vi "SDO_DRIVE_ACT.vi"(6 "Pass_Through_Time":dbl=-1.0 format="%33.4f", 8 "error in (no error)":errorcluster, 10 "Swerve Drive Device Reference":T1[](array[typedef])) -> (0 "error out":errorcluster)   [LabVIEW 2019]
uses:
  SDO_DRIVE_MODULE_TYPDEF.ctl
  <vilib>/Rock Robotics/WPI/MotorControl/WPI_MotorControlDeviceRef.ctl
  <vilib>/Rock Robotics/WPI/MotorControl/WPI_MotorControlType.ctl
  <vilib>/Rock Robotics/SystemInterfaces/DIO/FPGA_DIOPWMChannel.ctl
  <vilib>/Rock Robotics/WPI/PWM/WPI_PWMDeadband.ctl
  <vilib>/Rock Robotics/SystemInterfaces/DIO/FPGA_DIOChannel.ctl
  <vilib>/Rock Robotics/WPI/Encoder/WPI_EncoderDevRef.ctl
  <vilib>/Rock Robotics/SystemInterfaces/Encoder/FPGA_EncoderIdx.ctl
  <vilib>/Rock Robotics/SystemInterfaces/Counter/FPGA_CounterCtrSystemIndex.ctl
  <vilib>/Rock Robotics/WPI/Encoder/WPI_EncoderType.ctl
  <vilib>/Rock Robotics/WPI/ThirdParty/JAS_Junk/TrajLib/VI/numCmd_Recv_Generic.vi
  <vilib>/Rock Robotics/WPI/ThirdParty/JAS_Junk/TrajLib/VI/Util_GetTime_U32.vi
  <vilib>/Rock Robotics/WPI/ThirdParty/JAS_Junk/TrajLib/VI/numCmd_ObtainQueue_Generic.vi
  SDO_DRIVE_GLOBALS.vi
  <vilib>/Rock Robotics/WPI/ThirdParty/JAS_Junk/TrajLib/VI/Util_GetTime_U64.vi
  <vilib>/Rock Robotics/WPI/ThirdParty/JAS_Junk/TrajLib/Trajectory_Library.lvlib
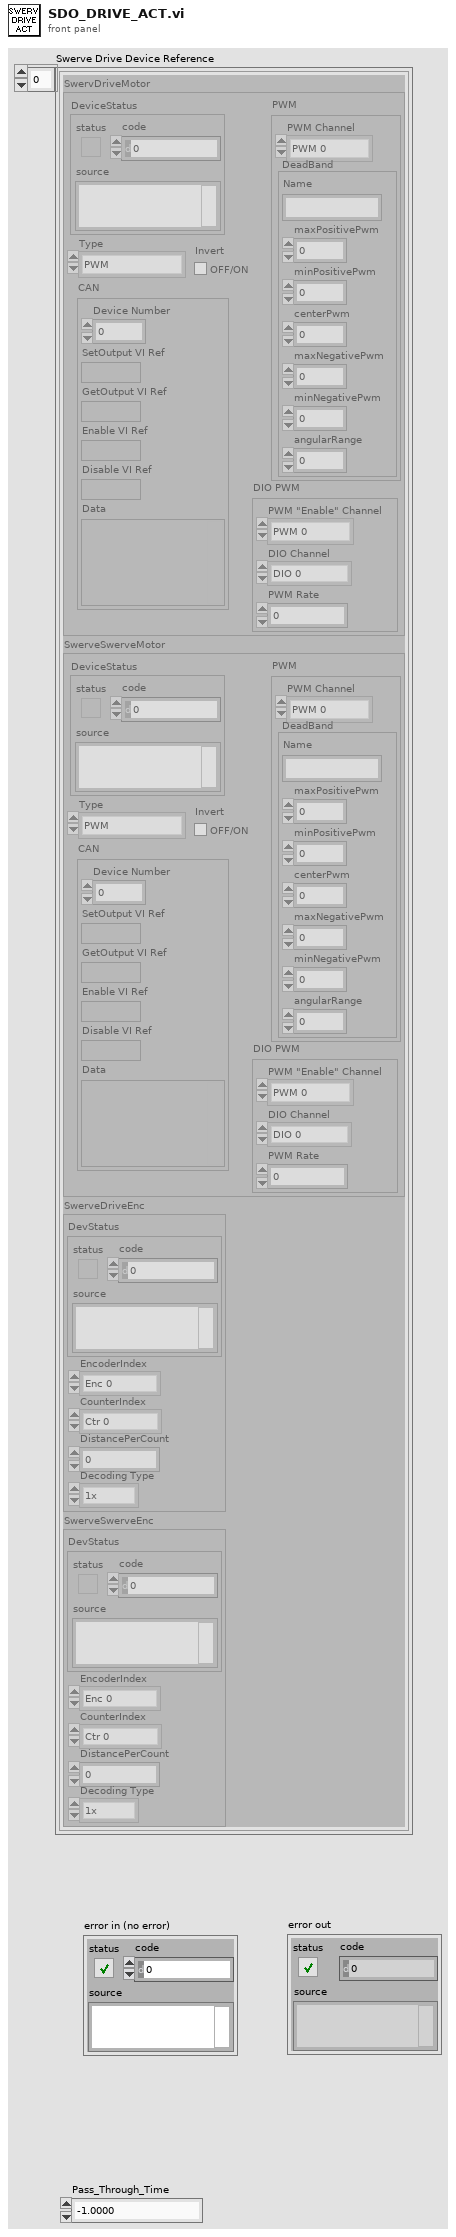
[diagram p1: front panel]
types:
  T1 = typedef "SDO_DRIVE_MODULE_TYPDEF.ctl" = cluster{"SwervDriveMotor":T2, "SwerveSwerveMotor":T2, "SwerveDriveEnc":T7, "SwerveSwerveEnc":T7}
  T2 = typedef "WPI_MotorControlDeviceRef.ctl" = cluster{"DeviceStatus":errorcluster, "Type":T3, "PWM":cluster{"PWM Channel":T4, "DeadBand":T5}, "CAN":cluster{"Device Number":u8, "SetOutput VI Ref":variant, "GetOutput VI Ref":variant, "Enable VI Ref":variant, "Disable VI Ref":variant, "Data":variant}, "Invert":bool, "DIO PWM":cluster{"PWM \"Enable\" Channel":T4, "DIOChannel":T6, "PWM Rate":dbl}}
  T3 = typedef "WPI_MotorControlType.ctl" = enum16{"PWM", "CAN", "DIO PWM"}
  T4 = typedef "FPGA_DIOPWMChannel.ctl" = enum8{"PWM 0", "PWM 1", "PWM 2", "PWM 3", "PWM 4", "PWM 5", "PWM 6", "PWM 7", "PWM 8", "PWM 9", "PWM MXP 0", "PWM MXP 1", "PWM MXP 2", "PWM MXP 3", "PWM MXP 4", "PWM MXP 5", "PWM MXP 6", "PWM MXP 7", "PWM MXP 8", "PWM MXP 9", "Invalid"}
  T5 = typedef "WPI_PWMDeadband.ctl" = cluster{"Name":string, "maxPositivePwm":i32, "minPositivePwm":i32, "centerPwm":i32, "maxNegativePwm":i32, "minNegativePwm":i32, "angularRange":u16}
  T6 = typedef "FPGA_DIOChannel.ctl" = enum8{"DIO 0", "DIO 1", "DIO 2", "DIO 3", "DIO 4", "DIO 5", "DIO 6", "DIO 7", "DIO 8", "DIO 9", "DIO MXP 0", "DIO MXP 1", "DIO MXP 2", "DIO MXP 3", "DIO MXP 4", "DIO MXP 5", "DIO MXP 6", "DIO MXP 7", "DIO MXP 8", "DIO MXP 9", "DIO MXP 10", "DIO MXP 11", "DIO MXP 12", "DIO MXP 13", "DIO MXP 14", "DIO MXP 15", "SPI Port CS1", "SPI Port CS2", "SPI Port CS3", "SPI Port MISO", "SPI Port MOSI", "Invalid"}
  T7 = typedef "WPI_EncoderDevRef.ctl" = cluster{"DevStatus":errorcluster, "EncoderIndex":T8, "CounterIndex":T9, "DistancePerCount":dbl, "Decoding Type":T10}
  T8 = typedef "FPGA_EncoderIdx.ctl" = enum8{"Enc 0", "Enc 1", "Enc 2", "Enc 3", "Enc 4", "Enc 5", "Enc 6", "Enc 7", "Invalid"}
  T9 = typedef "FPGA_CounterCtrSystemIndex.ctl" = enum8{"Ctr 0", "Ctr 1", "Ctr 2", "Ctr 3", "Ctr 4", "Ctr 5", "Ctr 6", "Ctr 7", "Invalid"}
  T10 = typedef "WPI_EncoderType.ctl" = enum16{"1x", "2x", "4x"}
  T11 = typedef "Trajectory_Library.lvlib/SWERVE_DRIVE_KINEMATICS.ctl" = cluster{"NumModules":i32, "InverseKinematics":T12, "ForwardKinematics":T12, "Modules":T13[], "PrevCoR":T13, "SavedModuleStates":T14[]}
  T12 = typedef "NI_Matrix.lvlib/RealMatrix.ctl" = dbl[][]
  T13 = typedef "Trajectory_Library.lvlib/TRANSLATION2D.ctl" = cluster{"X":dbl, "Y":dbl}
  T14 = typedef "Trajectory_Library.lvlib/SWERVE_DRIVE_MODULE_STATE.ctl" = cluster{"Speed":dbl, "Angle":T15}
  T15 = typedef "Trajectory_Library.lvlib/ROTATION2D.ctl" = cluster{"VALUE":dbl, "COS":dbl, "SIN":dbl}
  T16 = typedef "Trajectory_Library.lvlib/CHASSIS_SPEEDS.ctl" = cluster{"vX":dbl, "vY":dbl, "vOmega":dbl}
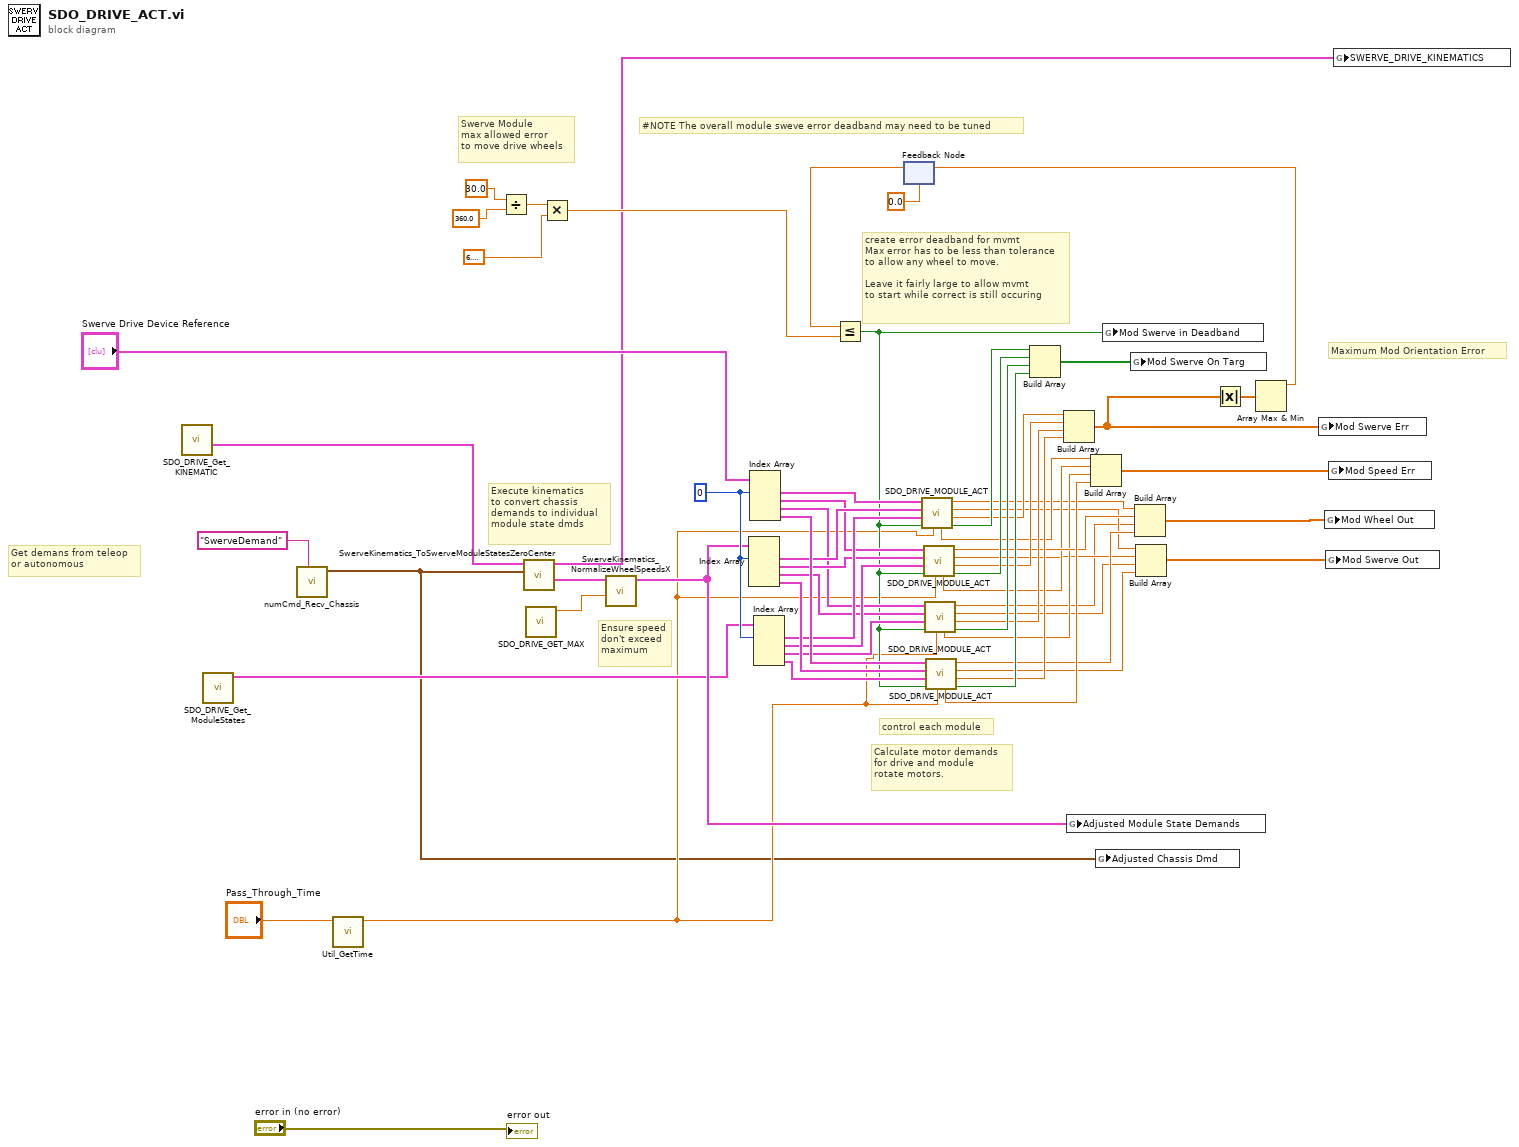
[diagram p0: block diagram]
diagram:
  w33 = 0 ("index")
  # "Swerve Module\nmax allowed error\nto move drive wheels"
  # "Ensure speed\ndon't exceed\nmaximum"
  # "Maximum Mod Orientation Error"
  # "#NOTE The overall module sweve error deadband may need to be tuned"
  # "create error deadband for mvmt\nMax error has to be less than tolerance\nto allow any wheel to move. \n\nLeave it fairly large to allow mvmt\nto start while correct is still occuring"
  # "Calculate motor demands\nfor drive and module \nrotate motors."
  # "Execute kinematics\nto convert chassis \ndemands to individual\nmodule state dmds"
  # "Get demans from teleop\nor autonomous"
  # "control each module"
  n1 = call "SDO_DRIVE_Get_KINEMATIC.vi"() -> ("out SWERVE_DRIVE_KINEMATICS"=w7:T11)  [unwired: 11 in]
  n2 = call "SDO_DRIVE_Get_ModuleStates.vi"() -> ("Swerve Module States"=w6:T14[])  [unwired: 11 in]
  n3 = call <vilib>:"numCmd_Recv_Chassis.vi"("Command Name"="SwerveDemand") -> ("Chassis Speeds"=w1:T16)  [unwired: 8 in, 2 out]
  n4 = call <vilib>:"Util_GetTime.vi"("Pass_Through_Time"="Pass_Through_Time") -> ("FPGA_Time_Seconds"=w3:dbl)  [unwired: 8 in, 2 out]
  n5 = Divide(x=30.0, y=360.0) -> (x/y=w56:dbl)
  n6 = call <vilib>:"SwerveKinematics_ToSwerveModuleStatesZeroCenter.vi"("ChassisSpeeds"=w1, "in SWERVE_DRIVE_KINEMATICS"=w7) -> ("ModuleStates"=w16:T14[], "out SWERVE_DRIVE_KINEMATICS"=w4:T11)  [unwired: 8 in]
  n7 = call "SDO_DRIVE_GET_MAX.vi"() -> ("Max Wheel Vel (Meter/Sec)"=w17:dbl)  [unwired: 10 in, 1 out]
  n8 = Multiply(x=w56, y=6.283185307179586) -> (x*y=w60:dbl)
  n9 = call <vilib>:"SwerveKinematics_NormalizeWheelSpeedsX.vi"("AttainableMaxSpeed"=w17, "in WheelStates"=w16) -> ("out WheelStates"=w8:T14[])  [unwired: 9 in]
  n10 = Index Array(array=w8, index #1=w33) -> (element #1=w22:T14, element #2=w23:T14, element #3=w24:T14, element #4=w37:T14)  [unwired: 3 in]
  n11 = Index Array(array="Swerve Drive Device Reference", index #1=w33) -> (element #1=w19:T1, element #2=w20:T1, element #3=w21:T1, element #4=w36:T1)  [unwired: 3 in]
  n12 = Index Array(array=w6, index #1=w33) -> (element #1=w25:T14, element #2=w26:T14, element #3=w27:T14, element #4=w38:T14)  [unwired: 3 in]
  n13 = feedback #1(0.0) -> (w55:dbl)
  n14 = Less Or Equal?(x=w55, y=w60) -> (x <= y?=w11:bool)
  n15 = call "SDO_DRIVE_MODULE_ACT.vi"("Pass_Through_Time"=w3, "SwervePosInDeadband"=w11, "Swerve State"=w25, "Swerve Dmd"=w22, "Swerve Module TypDef"=w19) -> ("SwerveOnTarget"=w48:bool, "SwervePosError"=w43:dbl, "Swerve Motor Dmd"=w30:dbl, "Wheel Motor Dmd"=w28:dbl, "WheelSpeedErr"=w39:dbl)  [unwired: 2 in]
  n16 = call "SDO_DRIVE_MODULE_ACT.vi"("Pass_Through_Time"=w3, "SwervePosInDeadband"=w11, "Swerve State"=w26, "Swerve Dmd"=w23, "Swerve Module TypDef"=w20) -> ("SwerveOnTarget"=w49:bool, "SwervePosError"=w44:dbl, "Swerve Motor Dmd"=w31:dbl, "Wheel Motor Dmd"=w42:dbl, "WheelSpeedErr"=w40:dbl)  [unwired: 2 in]
  n17 = call "SDO_DRIVE_MODULE_ACT.vi"("Pass_Through_Time"=w3, "SwervePosInDeadband"=w11, "Swerve State"=w27, "Swerve Dmd"=w24, "Swerve Module TypDef"=w21) -> ("SwerveOnTarget"=w50:bool, "SwervePosError"=w45:dbl, "Swerve Motor Dmd"=w32:dbl, "Wheel Motor Dmd"=w29:dbl, "WheelSpeedErr"=w41:dbl)  [unwired: 2 in]
  n18 = call "SDO_DRIVE_MODULE_ACT.vi"("Pass_Through_Time"=w3, "SwervePosInDeadband"=w11, "Swerve State"=w38, "Swerve Dmd"=w37, "Swerve Module TypDef"=w36) -> ("SwerveOnTarget"=w51:bool, "SwervePosError"=w46:dbl, "Swerve Motor Dmd"=w35:dbl, "Wheel Motor Dmd"=w34:dbl, "WheelSpeedErr"=w47:dbl)  [unwired: 2 in]
  n19 = Build Array(w48, w49, w50, w51) -> (w10:bool[])
  n20 = Build Array(w43, w44, w45, w46) -> (w13:dbl[])
  n21 = global write "SDO_DRIVE_GLOBALS.vi" "Adjusted Module State Demands"(w8) -> ()
  n22 = Build Array(w39, w40, w41, w47) -> (w12:dbl[])
  n23 = global write "SDO_DRIVE_GLOBALS.vi" "Adjusted Chassis Dmd"(w1) -> ()
  n24 = global write "SDO_DRIVE_GLOBALS.vi" "Mod Swerve in Deadband"(w11) -> ()
  n25 = global write "SDO_DRIVE_GLOBALS.vi" "Mod Swerve On Targ"(w10) -> ()
  n26 = Build Array(w28, w42, w29, w34) -> (w15:dbl[])
  n27 = Build Array(w30, w31, w32, w35) -> (w14:dbl[])
  n28 = Absolute Value(x=w13) -> (abs(x)=w52:dbl[])
  n29 = Array Max & Min(array=w52) -> (max value=w53:dbl)  [unwired: 3 out]
  n30 = feedback-in #1(w53) -> ()
  n31 = global write "SDO_DRIVE_GLOBALS.vi" "Mod Swerve Err"(w13) -> ()
  n32 = global write "SDO_DRIVE_GLOBALS.vi" "Mod Wheel Out"(w15) -> ()
  n33 = global write "SDO_DRIVE_GLOBALS.vi" "Mod Swerve Out"(w14) -> ()
  n34 = global write "SDO_DRIVE_GLOBALS.vi" "Mod Speed Err"(w12) -> ()
  n35 = global write "SDO_DRIVE_GLOBALS.vi" "SWERVE_DRIVE_KINEMATICS"(w4) -> ()
  "error out" <- "error in (no error)"
